vi "LVH5Rdereference (DSet).vi"(6 "error in (no error)":errorcluster, 8 "HDF5 Dataset Region Ref":T2, 9 "HDF5 Dataset Ref":T1) -> (0 "error out":errorcluster, 2 "HDF5 Referred Dataset":T1, 3 "HDF5 Dataset Ref out":T1)   [LabVIEW 2017]
doc: "Opens the HDF5 object referenced."
uses:
  <vilib>/UPVI/lvhdf5/library.llb/HDF5 Ref.ctl
  <vilib>/UPVI/lvhdf5/reference.llb/H5R Dataset Region Ref.ctl
  <vilib>/UPVI/lvhdf5/h5helper.dll
panel:
  # "LVHDF5 Toolkit\nCopyright (c) 2005-2013 by Jason D. Sommerville\nCopyright (c) 2014 by UPVI, LLC.\n\nThis use and distribution of this file is governed by the terms found in \nLICENSE.txt distributed with this toolkit and installed at\n <user.lib>\\_lvhdf5\\LICENSE.txt"
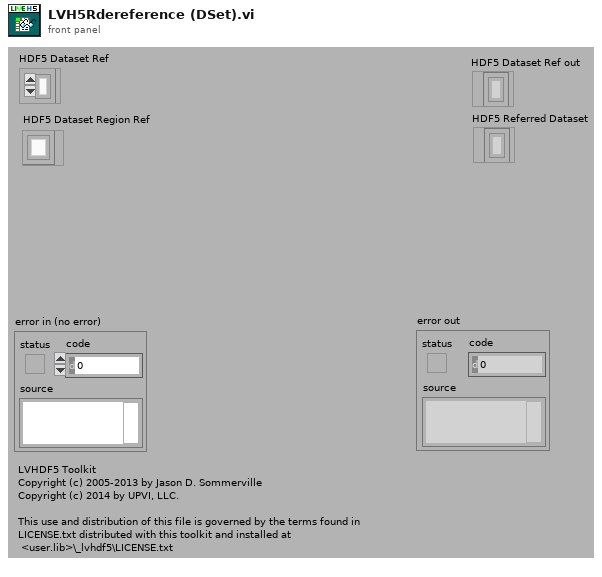
[diagram p1: front panel]
types:
  T1 = typedef "HDF5 Ref.ctl" = refnum<k1>
  T2 = typedef "H5R Dataset Region Ref.ctl" = refnum<k1>
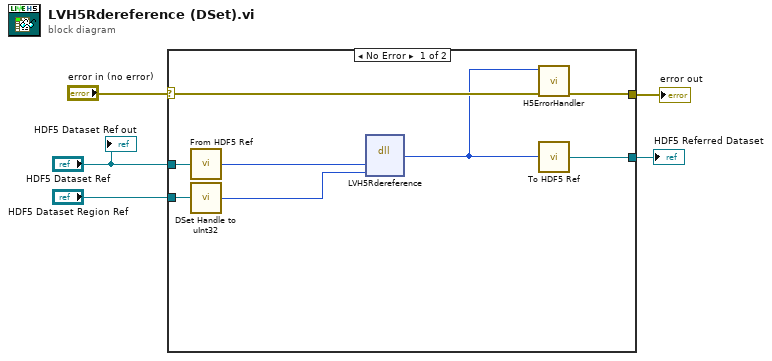
[diagram p0: block diagram]
diagram:
  n1 = case shown="No Error" "error in (no error)" {
    selector: "error in (no error)" -> [w13 w14]
    tunnel: [w12 w14] -> w4
    tunnel: "HDF5 Dataset Ref" -> [w11 _]
    tunnel: "HDF5 Dataset Region Ref" -> [w9 _]
    tunnel: [w6 _] -> w1
    frame No Error {
      n2 = call <vilib>:"From HDF5 Ref.vi"("HDF5 Ref"=w11) -> ("I32"=w10:i32)
      n3 = call <vilib>:"DSet Handle to uInt32.vi"("HDF5 Reference Type"=w9) -> ("Handle"=w8:u32)
      n4 = dll-call lib="C:/Program Files/National Instruments/LabVIEW 2017/vi.lib/UPVI/lvhdf5/h5helper.dll" fn="LVH5Rdereference"("dset_id"=w10, "handle"=w8) -> (w7:i32)  [unwired: 5 in, 2 out]
      n5 = call <vilib>:"H5ErrorHandler.vi"("error in (no error)"=w13, "herr_t"=w7) -> ("error out"=w12:errorcluster)  [unwired: 3 in, 4 out]
      n6 = call <vilib>:"To HDF5 Ref.vi"("I32"=w7) -> ("HDF5 Ref"=w6:T1)
    }
    frame Error {
    }
  }
  "error out" <- w4
  "HDF5 Referred Dataset" <- w1
  "HDF5 Dataset Ref out" <- "HDF5 Dataset Ref"
